vi "Key.vi"(8 "Error In":errorcluster, 11 "Token":refnum<class "Abstract.lvclass">) -> (0 "Error Out":errorcluster, 3 "Key":string)   [LabVIEW 2018, in "Toolkit.lvlib" / "Compiler.lvclass"]
uses:
  Compiler.lvclass
  Tokens/Abstract/Abstract.lvclass
  Tokens/Keyable/API/Keyable.lvclass
  Tokens/Keyable/API/Keyable.lvclass/Keyable.ctl
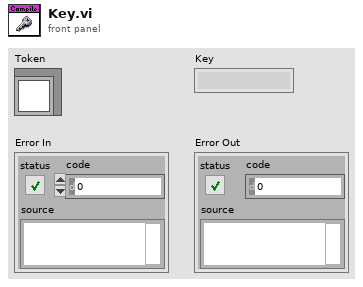
[diagram p1: front panel]
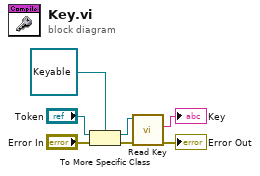
[diagram p0: block diagram]
diagram:
  n1 = To More Specific Class(target class=refnum<class "Keyable.lvclass"> refnum ("Toolkit.lvlib:Tokens.lvlib:Keyable.lvclass"), reference="Token", error in="Error In") -> (specific class reference=w4:refnum<class "Keyable.lvclass">, error out=w3:errorcluster)
  n2 = call "Read Key.vi"("Error In"=w3, "Keyable In"=w4) -> ("Error Out"=→"Error Out":errorcluster, "Key"=→"Key":string)  [unwired: 7 in, 1 out]
